vi "Common Receive.vi"(6 "W/R":enum16{"Write", "Read"}(ring), 7 "Data Type":T1=enum."U16", 8 "error in":errorcluster, 9 "Data":i64, 10 "PDO Name":string="Controlword", 11 "Motor Base in":refnum<class "Motor Base.lvclass">) -> (0 "error out":errorcluster, 2 "Data":i64, 3 "Motor Base out":refnum<class "Motor Base.lvclass">)   [LabVIEW 2016, in "Motor Base.lvlib" / "Motor Base.lvclass"]
uses:
  Motor Base.lvclass
  Data Type.ctl
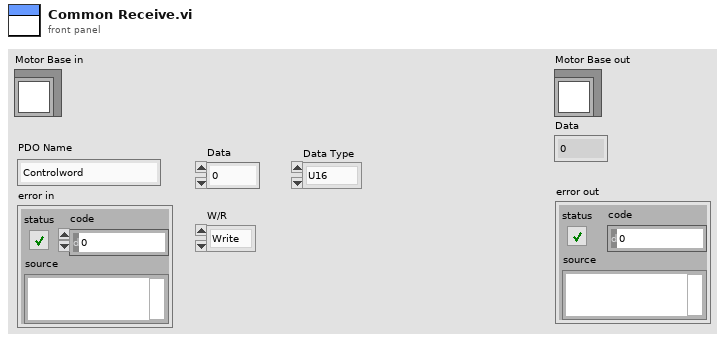
[diagram p1: front panel]
types:
  T1 = typedef "Motor Base.lvlib/Motor Base.lvclass/Data Type.ctl" = enum16{"BOOL", "I16", "I32", "I8", "OS", "U16", "U32", "U8", "VS"}
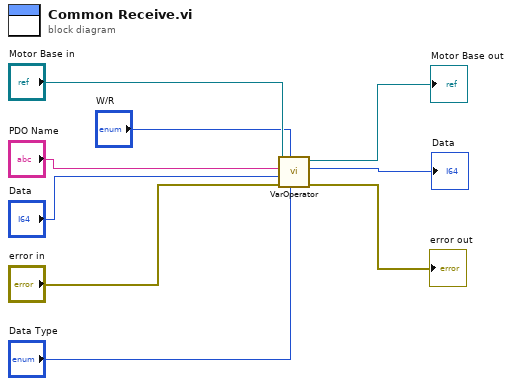
[diagram p0: block diagram]
diagram:
  n1 = call-dynamic "VarOperator.vi"("Data Type"="Data Type", "ro/w/r"="W/R", "error in"="error in", "Data"="Data", "PDO Name"="PDO Name", "Motor Base in"="Motor Base in") -> ("error out"=→"error out":errorcluster, "Data"=→"Data":i64, "Motor Base out"=→"Motor Base out":refnum<class "Motor Base.lvclass">)  [unwired: 1 in, 2 out]
